vi "Read To String_True.vi"(8 "error in (no error)":errorcluster, 11 "Abs_Boolean_1D in":refnum<class "Abs_Boolean_1D.lvclass">) -> (0 "error out":errorcluster, 2 "To String:True":string="True", 3 "Abs_Boolean_1D out":refnum<class "Abs_Boolean_1D.lvclass">)   [LabVIEW 2021, in "Abs_Boolean_1D.lvclass"]
uses:
  Abs_Boolean_1D.lvclass
  Abs_Boolean_1D.lvclass/Abs_Boolean_1D.ctl
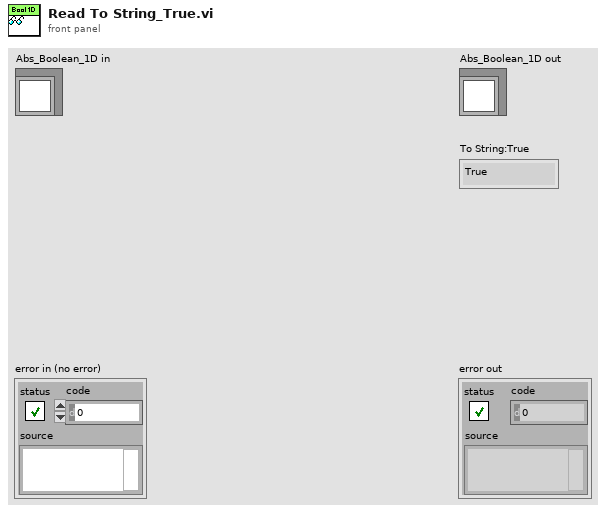
[diagram p1: front panel]
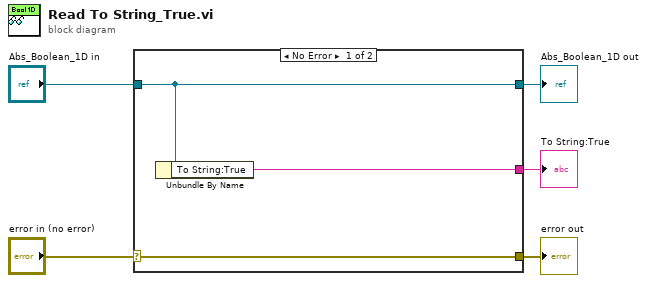
[diagram p0: block diagram]
diagram:
  n1 = case shown="No Error" "error in (no error)" {
    selector: "error in (no error)" -> [w8 w9]
    tunnel: [w8 w9] -> w4
    tunnel: [w7 w10] -> w2
    tunnel: "Abs_Boolean_1D in" -> [w7 w10]
    tunnel: [w6 _] -> w1
    frame No Error {
      n2 = Unbundle By Name(w7) -> ("To String:True"=w6:string)
    }
    frame Error {
    }
  }
  "error out" <- w4
  "Abs_Boolean_1D out" <- w2
  "To String:True" <- w1
